vi "RT Channel List FGV.vi"(7 "Enum":enum16{"Read", "Write"}(ring), 8 "error in (no error)":errorcluster, 11 "Channel List in":T1) -> (0 "error out":errorcluster, 3 "Channel List":T1)   [LabVIEW 2022 SP3]
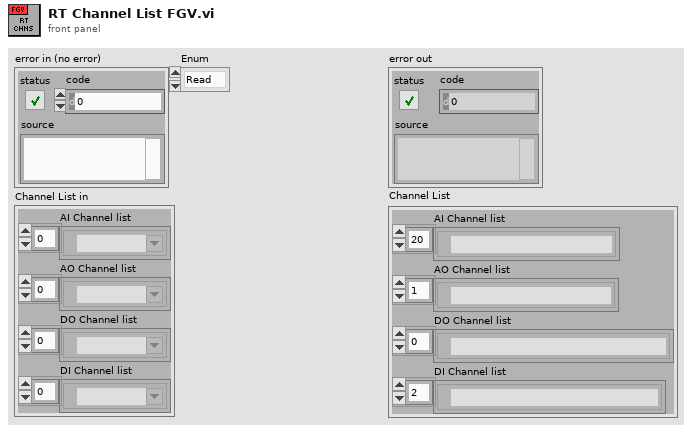
[diagram p1: front panel]
types:
  T1 = cluster{"AI Channel list":tag[], "AO Channel list":tag[], "DO Channel list ":tag[], "DI Channel list":tag[]}
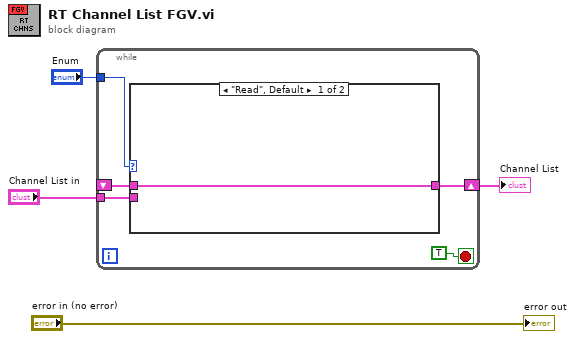
[diagram p0: block diagram]
diagram:
  n1 = while {
    tunnel: "Enum" -> [w8]
    shift-right: [w9] -> w4
    shift-left: _ -> [w7]
    tunnel: "Channel List in" -> [w5]
    stop <- TRUE stop-if-true
    n2 = case shown="\"Read\", Default" w8 {
      tunnel: [w10 w11] -> w9
      tunnel: w7 -> [w10 _]
      tunnel: w5 -> [_ w11]
      frame "Read", Default {
      }
      frame "Write" {
      }
    }
  }
  "Channel List" <- w4
  "error out" <- "error in (no error)"
